vi "Set Target ID.vi"(8 "target ID":string, 11 "instVIref":T1) -> (3 "instVIref out":T1)   [LabVIEW 2020, in "NI_TargetHelper.lvlib"]
uses:
  <vilib>/TargetSupport/NI_TargetHelper/NI_TargetHelper.lvlib
  <vilib>/TargetSupport/NI_TargetHelper/Instance VIref.ctl
  <vilib>/UserTags/UserTags.lvlib
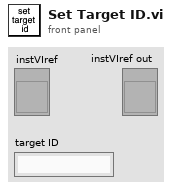
[diagram p1: front panel]
types:
  T1 = typedef "NI_TargetHelper.lvlib/Instance VIref.ctl" = refnum<vi>
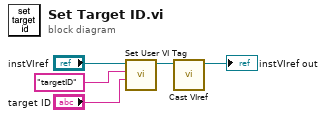
[diagram p0: block diagram]
diagram:
  n1 = call <vilib>:"Set User VI Tag.vi"("Value"="target ID", "Tag Name"="targetID", "VI Refnum"="instVIref") -> ("dup VI Refnum"=w3:refnum<vi>)  [unwired: 6 in, 2 out]
  n2 = call <vilib>:"Cast VIref.vi"("VI Refnum"=w3) -> ("instVIref"=→"instVIref out":T1)  [unwired: 10 in]
